vi "Pre Launch Init.vi"(11 "ExampleSimpleRootModel in":refnum<class "SimpleRootModel.lvclass">) -> (0 "error out":errorcluster, 3 "ExampleSimpleRootModel out":refnum<class "SimpleRootModel.lvclass">)   [LabVIEW 2020, in "MVAExamples.lvlib" / "SimpleRootModel.lvclass"]
doc: "(<B>Filename</B>: Actor Framework.lvlib:Actor.lvclass:Pre Launch Init.vi)\n\nDefines behavior that occurs after the Launch Nested Actor method is invoked but before the actor's Actor Core method begins running.\n\nBy default, this method does nothing. A descendant class may override it to define behavior."
uses:
  SimpleRootModel.lvclass
  C:/Program Files/National Instruments/LabVIEW 2020/vi.lib/ActorFramework/Actor/Actor.lvclass
  <vilib>/ActorFramework/Actor/Actor.lvclass/Actor.ctl
  <vilib>/ActorFramework/Message Enqueuer/Message Enqueuer.lvclass/Message Enqueuer.ctl
  modules/mva-core/Source/SubscriptionPolicy/ValueChangeSubscription/ValueChangeSubscription.lvclass/ValueChangeSubscription.ctl
  modules/mva-core/Source/IObserver/IObserver Messages/Observe Data Msg/Observe Data Msg.lvclass/Observe Data Msg.ctl
  modules/composed-af-messages/Source/RoundTripMessage/RoundTripMessage.lvclass/RoundTripMessage.ctl
  modules/mva-core/Source/IObserver/ActorDataBinding/ActorDataBinding.lvclass/ActorDataBinding.ctl
  modules/mva-core/Source/IMediator/SubscriptionRequest/SubscriptionRequest.lvclass/SubscriptionRequest.ctl
  modules/mva-core/Source/IObserver/IObserver Messages/Subscribe Msg/Subscribe Msg.lvclass/Subscribe Msg.ctl
  SimpleRootModel.lvclass/SimpleRootModel.ctl
  ExampleSimpleRootModel Messages/Execute State Msg/Execute State Msg.lvclass/Execute State Msg.ctl
  modules/mva-core/Source/IMediator/SubscriptionRequest/Pack Subscription Request.vi
  modules/mva-core/Source/SubscriptionPolicy/BasicSubscription/New Basic Subscription.vi
  modules/mva-core/Source/SubscriptionPolicy/ValueChangeSubscription/New Value Change Subscription.vi
  modules/mva-core/Source/IObserver/ActorDataBinding/New Actor Data Binding Transport.vi
  modules/mva-core/Source/IObserver/IObserver Messages/Subscribe Msg/Send Subscribe.vi
  <vilib>/ActorFramework/Message Enqueuer/Init from Existing Queue.vi
  <vilib>/ActorFramework/Message Enqueuer/Enqueue.vi
  modules/mva-core/Source/IObserver/IObserver Messages/Observe Data Msg/Write Observe Data Msg Return Info.vi
  modules/composed-af-messages/Source/RoundTripMessage/Write Return Address.vi
  modules/mva-core/Source/SubscriptionPolicy/ValueChangeSubscription/ValueChangeSubscription.lvclass
  modules/mva-core/Source/IObserver/IObserver/IObserver.lvclass
  modules/mva-core/Source/IObserver/IObserver Messages/Observe Data Msg/Observe Data Msg.lvclass
  modules/mva-core/Source/IObserver/ActorDataBinding/ActorDataBinding.lvclass
  modules/mva-core/Source/IObserver/IObserver Messages/Subscribe Msg/Subscribe Msg.lvclass
  C:/Program Files/National Instruments/LabVIEW 2020/vi.lib/ActorFramework/Message/Message.lvclass
  ExampleSimpleRootModel Messages/Execute State Msg/Execute State Msg.lvclass
  modules/mva-core/Source/IMediator/ISubscriptionPolicy/Open Subscription Policy.vi
  <vilib>/Utility/error.llb/Error Cluster From Error Code.vi
  <vilib>/ActorFramework/Message Priority Queue/Priority Enqueue.vi
  modules/mva-core/Source/IModel/IModel/IModel.lvclass
  modules/mva-core/Source/SubscriptionPolicy/BasicSubscription/BasicSubscription.lvclass
  <vilib>/ActorFramework/Message Enqueuer/Message Enqueuer.lvclass
  modules/mva-core/Source/IMediator/SubscriptionRequest/SubscriptionRequest.lvclass
  <vilib>/ActorFramework/Actor/Actor.lvclass
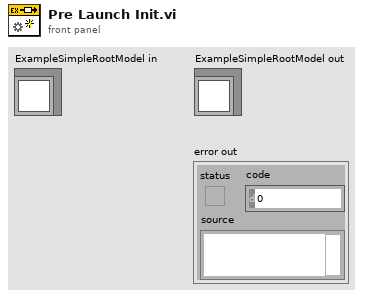
[diagram p1: front panel]
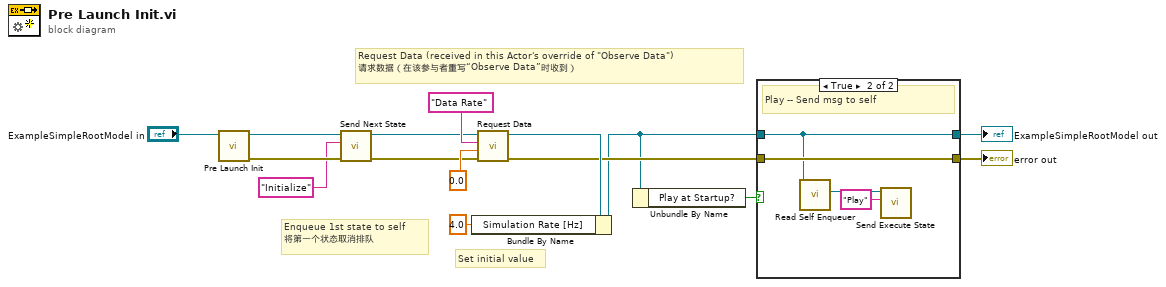
[diagram p0: block diagram]
diagram:
  # "Request Data (received in this Actor's override of \"Observe Data\")\n请求数据（在该参与者重写“Observe Data”时收到）"
  # "Set initial value"
  # "Enqueue 1st state to self\n将第一个状态取消排队"
  n1 = call-parent "Pre Launch Init.vi"("IModel in"="ExampleSimpleRootModel in") -> ("error out"=w15:errorcluster, "IModel out"=w13:refnum<class "SimpleRootModel.lvclass">)  [unwired: 9 in]
  n2 = call "Send Next State.vi"("error in (no error)"=w15, "State"="Initialize", "ExampleSimpleRootModel in"=w13) -> ("error out"=w6:errorcluster, "ExampleSimpleRootModel out"=w7:refnum<class "SimpleRootModel.lvclass">)  [unwired: 7 in]
  n3 = call "Request Data.vi"("error in (no error)"=w6, "Data Type"=0.0, "Datum Name"="Data Rate", "IObserver in"=w7) -> ("error out"=w4:errorcluster, "IObserver out"=w11:refnum<class "SimpleRootModel.lvclass">)  [unwired: 5 in, 1 out]
  n4 = Bundle By Name(cluster=w11, "Simulation Rate [Hz]"=4.0) -> (w3:refnum<class "SimpleRootModel.lvclass">)
  n5 = Unbundle By Name(w3) -> ("Play at Startup?"=w5:bool)
  n6 = case shown="True" w5 {
    tunnel: w4 -> [w16 w21]
    tunnel: w3 -> [w17 w20]
    tunnel: [w17 w20] -> w2
    tunnel: [w16 w21] -> w1
    frame False {
      # "Wait for external msg"
      # "Do nothing"
    }
    frame True {
      # "Play -- Send msg to self"
      n7 = call <vilib>:"Read Self Enqueuer.vi"("Actor"=w20) -> ("Self Enqueuer"=w19:refnum<class "Message Enqueuer.lvclass">)  [unwired: 10 in]
      n8 = call "Send Execute State.vi"("State"="Play", "Message Enqueuer"=w19) -> ()  [unwired: 8 in, 2 out]
    }
  }
  "error out" <- w1
  "ExampleSimpleRootModel out" <- w2
